vi "LINX - PmodALS.vi"() -> ()   [LabVIEW 2019]
doc: "PmodALS\n\nThis example demonstrates how to read the relative light sensed from the PmodALS.\n\nInstructions:\n1. Select the COM Port associated with the LINX device\n2. Select the SPI Channel that the Pmod is connected to.\n3. Select the CS Channel that the Pmod is connected to.\n4. Click the Run Arrow."
uses:
  <vilib>/MakerHub/LINX/LMH-LINX.lvlib
  <vilib>/MakerHub/LINX/Public/Sensors/Pmods/ALS/PmodALS.lvlib
panel:
  in  "SPI Channel (0)":u8
  in  "Serial Port":refnum<visa-resource-name>="N/A"
  in  "CS Channel":u8=10
  out "Light Level (%)":dbl
  in  "Stop Button":bool
  # "PmodALS\n\nThis example demonstrates how to read the relative light \nsensed by the PmodALS.\n\nInstructions:\n1. Select the COM Port associated with the LINX device\n2. Select the SPI Channel that the Pmod is connected to.\n3. Select the CS Channel that the Pmod is connected to.\n4. Click the Run Arrow."
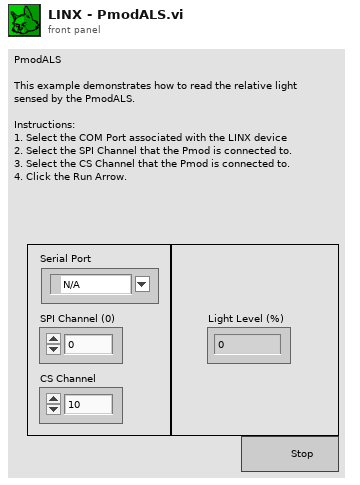
[diagram p1: front panel]
types:
  T1 = typedef "LMH-LINX.lvlib/LINX Ref.ctl" = cluster{"IO":T2, "Interface":T3, "LINX Device Config":T4}
  T2 = typedef "LMH-LINX.lvlib/Platform.ctl" = enum16{"Remote", "Local"}
  T3 = typedef "LMH-LINX.lvlib/Interface.ctl" = enum16{"Serial", "TCP"}
  T4 = typedef "LMH-LINX.lvlib/Device.lvlib/LINX Device Config.ctl" = cluster{"Interface":T3, "COM Port":refnum<visa-resource-name>, "TCP Configuration":T5, "Device Family":u8, "Device ID":u8, "Device Name":string, "TCP Ref":refnum<k5>, "Channels":T6}
  T5 = typedef "LMH-LINX.lvlib/Device.lvlib/TCP Config.ctl" = cluster{"IP Address":string, "Port":u16}
  T6 = typedef "LMH-LINX.lvlib/Channels.ctl" = cluster{"DI":u8[], "DO":u8[], "AI":u8[], "AO":u8[], "PWM":u8[], "QE":u8[], "UART":u8[], "I2C 2":u8[], "SPI":u8[], "CAN":u8[], "Servo":u8[], "AI Ref (V)":dbl, "AI Resolution (Bits)":u8, "AO Ref (V)":dbl, "AO Resolution (Bits)":u8}
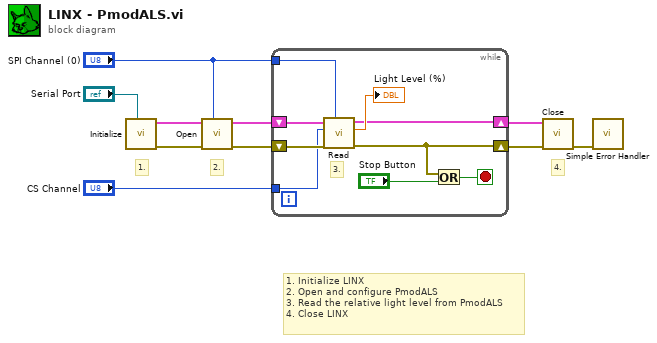
[diagram p0: block diagram]
diagram:
  # "4."
  # "1. Initialize LINX\n2. Open and configure PmodALS\n3. Read the relative light level from PmodALS\n4. Close LINX"
  # "2."
  # "1."
  n1 = call <vilib>:"Initialize.vi"("Serial Port"="Serial Port") -> ("Error Out"=w8:errorcluster, "LINX Resource"=w9:T1)  [unwired: 8 in, 1 out]
  n2 = call <vilib>:"Open.vi"("SPI Channel (0)"="SPI Channel (0)", "Error In"=w8, "LINX Resource"=w9) -> ("Error Out"=w6:errorcluster, "LINX Resource"=w7:T1)  [unwired: 7 in]
  n3 = while {
    shift-right: [w16] -> w4
    shift-left: w7 -> [w18]
    shift-right: [w11] -> w3
    shift-left: w6 -> [w17]
    tunnel: "CS Channel" -> [w15]
    tunnel: "SPI Channel (0)" -> [w14]
    stop <- w13 stop-if-true
    # "3."
    n4 = call <vilib>:"Read.vi"("SPI Channel (0)"=w14, "Error In"=w17, "CS Channel"=w15, "LINX Resource"=w18) -> ("Erro Out"=w11:errorcluster, "Light Level (%)"=→"Light Level (%)":dbl, "LINX Resource"=w16:T1)  [unwired: 5 in]
    n5 = Or(x=w11, y="Stop Button") -> (x .or. y?=w13:bool)
  }
  n6 = call <vilib>:"Close.vi"("Error In"=w3, "LINX Resource"=w4) -> ("Error Out"=w5:errorcluster)  [unwired: 9 in]
  n7 = call <vilib>:"Simple Error Handler.vi"("error in (no error)"=w5) -> ()  [unwired: 4 in, 5 out]
